vi "Serialize.vi"(0 "object in":refnum<class "JSONJDP.lvclass">, 2 "outputs":variant[](array[variant]), 5 "error in (no error)":errorcluster) -> (14 "object out":refnum<class "JSONJDP.lvclass">, 16 "JSON":string, 19 "error out":errorcluster)   [LabVIEW 2018, in "JSONJDP.lvclass"]
uses:
  JSONJDP.lvclass
  138fae1c-fe3b-439f-bdf0-6b9cf2aa9fe8.vi
  98a3f0f0-3c6e-455c-842b-17d1b66bd090.vi
  <vilib>/JDP Science/JSONtext/Variant to JSON Text.vi
  <vilib>/ErrorRing/Error Ring.xnode
  <vilib>/JDP Science/JSONtext/LVClass Serializer/JSONtext LVClass Serializer.lvclass
  <vilib>/Utility/Data Type/NI_Data Type.lvlib
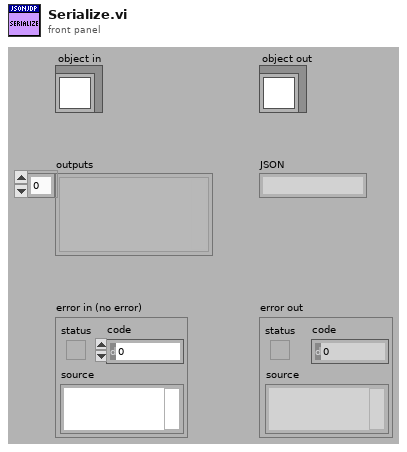
[diagram p1: front panel]
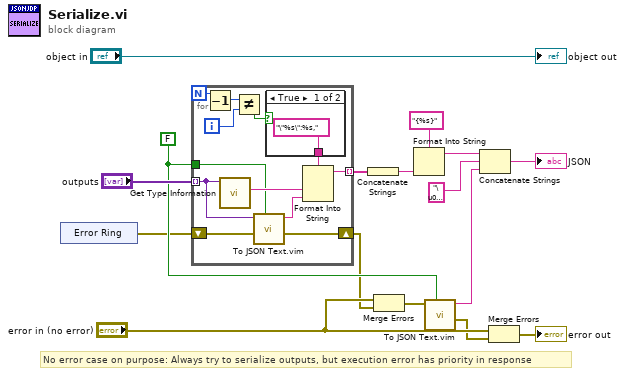
[diagram p0: block diagram]
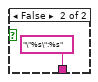
[diagram p2: hidden frame]
diagram:
  w4 = FALSE ("Multiline (T)")
  # "No error case on purpose: Always try to serialize outputs, but execution error has priority in response"
  n1 = xnode "Error Ring"() -> ("error out"=w2:errorcluster)
  n2 = for {
    N -> [w25]
    tunnel: "outputs" -> [w21] mode=indexing
    tunnel: [w26] -> w3 mode=indexing
    tunnel: w4 -> [w20]
    shift-right: [w18] -> w1
    shift-left: w2 -> [w17]
    i -> [w23]
    n3 = Decrement(x=w25) -> (x-1=w24:i32)
    n4 = call <vilib>:"Get Type Information.vi"("Variant"=w21) -> ("Name"=w27:string)  [unwired: 6 in, 4 out]
    n5 = Not Equal?(x=w24, y=w23) -> (x != y?=w22:bool)
    n6 = call "To JSON Text.vim"("enable LabVIEW extensions? (T)"=w20, "error in (no error)"=w17, "Anything"=w21) -> ("error out"=w18:errorcluster, "<JSON>"=w19:string)  [unwired: 7 in]
    n7 = case shown="True" w22 {
      tunnel: ["\"%s\":%s," ("format string") "\"%s\":%s" ("format string")] -> w28
      frame True {
      }
      frame False {
      }
    }
    n8 = Format Into String(format string=w28, w27, w19) -> (resulting string=w26:string)  [unwired: 2 in, 1 out]
  }
  n9 = Concatenate Strings(w3) -> (w14:string)
  n10 = Merge Errors("error in (no error)", w1) -> (w9:errorcluster)
  n11 = Format Into String(format string="{%s}", w14) -> (resulting string=w5:string)  [unwired: 2 in, 1 out]
  n12 = call "To JSON Text.vim"("enable LabVIEW extensions? (T)"=w4, "Anything"=w9) -> ("error out"=w8:errorcluster, "<JSON>"=w7:string)  [unwired: 8 in]
  n13 = Concatenate Strings(w5, "\u0017" ("Delimiter 3"), w7) -> (→"JSON":string)
  n14 = Merge Errors("error in (no error)", w8) -> (→"error out":errorcluster)
  "object out" <- "object in"
